vi "uv光源修改.vi"() -> ()   [LabVIEW 2018]
uses:
  <vilib>/Instr/_visa.llb/VISA Configure Serial Port (Instr).vi
panel:
  out "串口状态":bool
  out "错误输出":errorcluster
  in  "数值":u16
  in  "写入字符串":string="uvled"
  in  "光源强度":u16(ring) items=["5%", "10%", "15%", "20%", "25%", "30%", "40%", "45%", "50%", "55%", "60%", "65%", "70%", "75%", "80%", "85%", "90%", "95%", "100%", "开启光源", "关闭光源", "手动模式", "自动模式"]
  out "光源设置成功":bool
  in  "连接光源控制机":bool
  in  "发送":bool
  in  "停止":bool
  out "接收区":string
  out "连接成功":bool
  out "uv光源开启":bool
  out "uv光源关闭":bool
  in  "stop bits (10: 1 bit)":u16(ring)=10 caption="停止位（10: 1位）" items=["1.0"=10, "1.5"=15, "2.0"=20]
  in  "parity (0:none)":enum16{"None", "Odd", "Even", "Mark", "Space"}(ring) caption="奇偶（0:无）"
  in  "data bits (8)":u16=8 caption="数据比特(8)" min=5 max=8 step=1
  in  "baud rate (9600)":u32=9600 caption="波特率(9600)"
  in  "VISA resource name":refnum<visa-resource-name> caption="VISA资源名称"
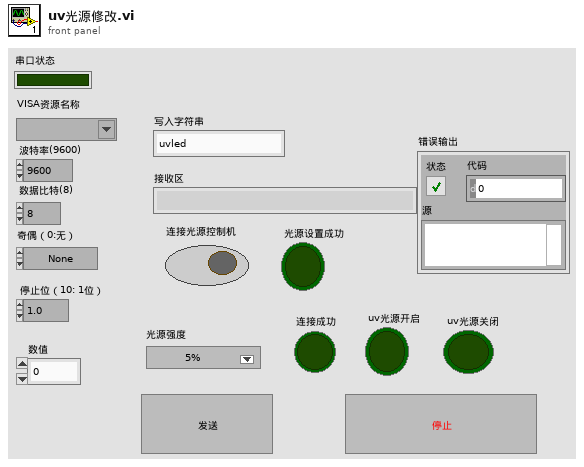
[diagram p1: front panel]
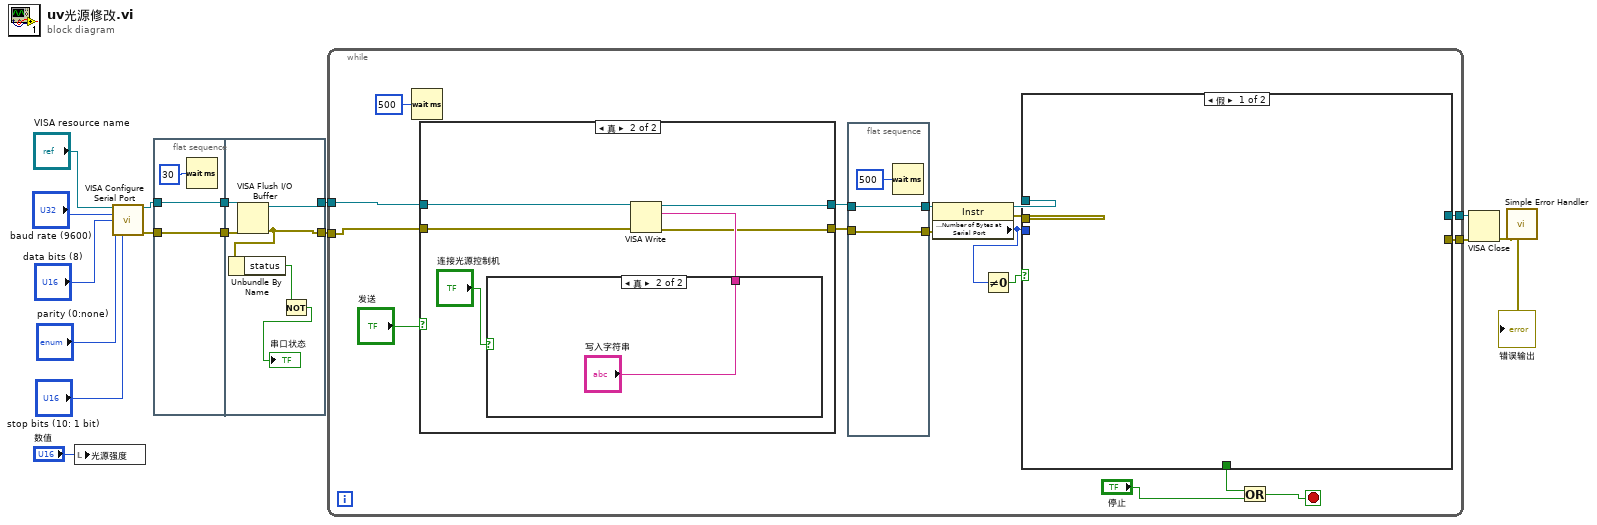
[diagram p0: block diagram]
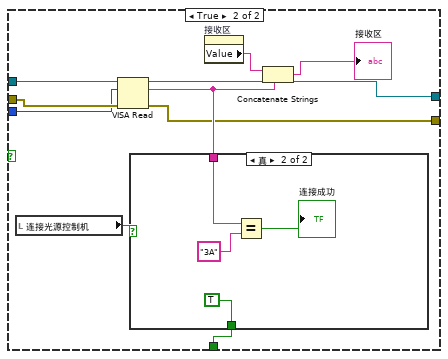
[diagram p2: hidden frame]
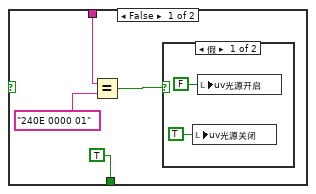
[diagram p3: hidden frame]
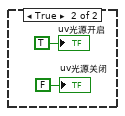
[diagram p4: hidden frame]
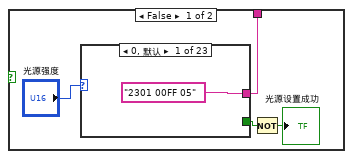
[diagram p6: hidden frame]
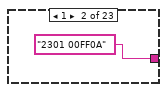
[diagram p7: hidden frame]
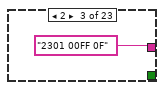
[diagram p8: hidden frame]
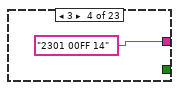
[diagram p9: hidden frame]
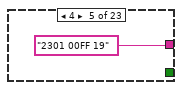
[diagram p10: hidden frame]
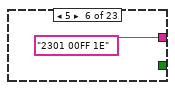
[diagram p11: hidden frame]
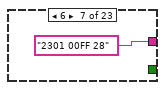
[diagram p12: hidden frame]
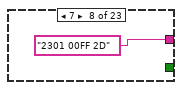
[diagram p13: hidden frame]
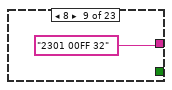
[diagram p14: hidden frame]
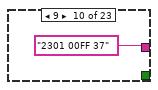
[diagram p15: hidden frame]
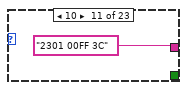
[diagram p16: hidden frame]
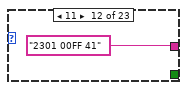
[diagram p17: hidden frame]
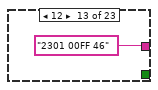
[diagram p18: hidden frame]
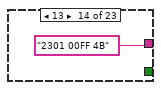
[diagram p19: hidden frame]
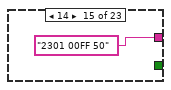
[diagram p20: hidden frame]
diagram:
  n1 = local write "光源强度"("数值") -> ()
  n2 = call-poly "VISA Configure Serial Port"("VISA resource name"="VISA resource name", "baud rate (9600)"="baud rate (9600)", "data bits (8)"="data bits (8)", "parity (0:none)"="parity (0:none)", "stop bits (10: 1 bit)"="stop bits (10: 1 bit)") -> ("VISA resource name out"=w4:refnum<visa-resource-name>, "error out"=w3:errorcluster)  [unwired: 9 in]
  n3 = flat-sequence {
    tunnel: w4 -> [w18]
    tunnel: w3 -> [w17]
    tunnel: [w18] -> w15
    tunnel: [w17] -> w14
    tunnel: [w21] -> w2
    tunnel: [w22] -> w1
    tunnel: w15 -> [w24]
    tunnel: w14 -> [w23]
    frame #0 {
      n4 = Wait (ms)(milliseconds to wait=u32 30 ("等待时间（毫秒）")) -> ()  [unwired: 1 out]
    }
    frame #1 {
      n5 = VISA Flush I/O Buffer(VISA resource name=w24, error in (no error)=w23) -> (VISA resource name out=w22:refnum<visa-resource-name>, error out=w21:errorcluster)  [unwired: 1 in]
      n6 = Unbundle By Name(w21) -> ("status"=w20:bool)
      n7 = Not(x=w20) -> (.not. x?=→"串口状态":bool)
    }
  }
  n8 = while {
    tunnel: w1 -> [w41]
    tunnel: [w29] -> w8
    tunnel: [w28] -> w6
    tunnel: w2 -> [w27]
    stop <- w32 stop-if-true
    n9 = Wait (ms)(milliseconds to wait=u32 500 ("等待时间（毫秒）")) -> ()  [unwired: 1 out]
    n10 = case shown="真" "发送" {
      tunnel: w41 -> [w67 w74]
      tunnel: w27 -> [w68 w73]
      tunnel: [w67 w71] -> w39
      tunnel: [w68 w70] -> w37
      frame False {
      }
      frame True {
        n11 = case shown="真" "连接光源控制机" {
          tunnel: [w78 "写入字符串"] -> w72
          frame False {
            n12 = case shown="0, 默认" "光源强度" {
              tunnel: ["2301 00FF 05" "2301 00FF0A" "2301 00FF 0F" "2301 00FF 14" "2301 00FF 19" "2301 00FF 1E" "2301 00FF 28" "2301 00FF 2D" "2301 00FF 32" "2301 00FF 37" "2301 00FF 3C" "2301 00FF 41" "2301 00FF 46" "2301 00FF 4B" "2301 00FF 50" "2301 00FF 55" "2301 00FF 5A" "2301 00FF 5F" "2301 00FF 64" "230E 0000 01" "230E 0000 00" "231E 00FF 03" "231E 00FF 01"] -> w78
              tunnel: [_ _ _ _ _ _ _ _ _ _ _ _ _ _ _ _ _ _ _ TRUE TRUE _ _] -> w76
              frame 0, Default {
              }
              frame 1 {
              }
              frame 2 {
              }
              frame 3 {
              }
              frame 4 {
              }
              frame 5 {
              }
              frame 6 {
              }
              frame 7 {
              }
              frame 8 {
              }
              frame 9 {
              }
              frame 10 {
              }
              frame 11 {
              }
              frame 12 {
              }
              frame 13 {
              }
              frame 14 {
              }
              frame 15 {
              }
              frame 16 {
              }
              frame 17 {
              }
              frame 18 {
              }
              frame 19 {
                # "开启光源"
              }
              frame 20 {
                # "关闭光源"
              }
              frame 21 {
                # "手动模式"
              }
              frame 22 {
                # "自动模式"
              }
            }
            n13 = Not(x=w76) -> (.not. x?=→"光源设置成功":bool)
          }
          frame True {
          }
        }
        n14 = VISA Write(VISA resource name=w74, write buffer=w72, error in (no error)=w73) -> (VISA resource name out=w71:refnum<visa-resource-name>, error out=w70:errorcluster)  [unwired: 1 out]
      }
    }
    n15 = flat-sequence {
      tunnel: w39 -> [w65]
      tunnel: [w65] -> w38
      tunnel: w37 -> [w64]
      tunnel: [w64] -> w36
      frame #0 {
        n16 = Wait (ms)(milliseconds to wait=u32 500 ("等待时间（毫秒）")) -> ()  [unwired: 1 out]
      }
    }
    n17 = property class="Instr"(reference=w38, error in=w36) -> (reference out=w34:refnum<visa-resource-name>, error out=w35:errorcluster, "Serial Settings:Number of Bytes at Serial Port"=w25:u32)
    n18 = Not Equal To 0?(x=w25) -> (x != 0?=w26:bool)
    n19 = case shown="假" w26 {
      tunnel: w35 -> [_ w51]
      tunnel: w34 -> [_ w50]
      tunnel: w25 -> [_ w49]
      tunnel: [_ w44] -> w31
      tunnel: [_ w43] -> w29
      tunnel: [_ w42] -> w28
      frame False {
      }
      frame True {
        n20 = local read "连接光源控制机"() -> (w46:bool)
        n21 = VISA Read(VISA resource name=w50, byte count=w49, error in (no error)=w51) -> (VISA resource name out=w42:refnum<visa-resource-name>, read buffer=w45:string, error out=w43:errorcluster)  [unwired: 1 out]
        n22 = case shown="真" w46 {
          tunnel: w45 -> [w55 w63]
          tunnel: [TRUE TRUE] -> w44
          frame False {
            n23 = Equal?(x=w55, y="240E 0000 01") -> (x = y?=w53:bool)
            n24 = case shown="假" w53 {
              frame False {
                n25 = local write "uv光源关闭"(TRUE ("uv光源关闭")) -> ()
                n26 = local write "uv光源开启"(FALSE ("uv光源开启")) -> ()
              }
              frame True {
                "uv光源开启" <- TRUE ("uv光源开启")
                "uv光源关闭" <- FALSE ("uv光源关闭")
              }
            }
          }
          frame True {
            n27 = Equal?(x=w63, y="3A") -> (x = y?=→"连接成功":bool)
          }
        }
        n28 = property on="接收区" class="Str"() -> ("Value"=w47:string)  [unwired: 2 in, 2 out]
        n29 = Concatenate Strings(w47, w45) -> (→"接收区":string)
      }
    }
    n30 = Or(x=w31, y="停止") -> (x .or. y?=w32:bool)
  }
  n31 = VISA Close(VISA resource name=w6, error in (no error)=w8) -> (error out=w7:errorcluster)
  "错误输出" <- w7
  n32 = call <vilib>:"Simple Error Handler.vi"("error in (no error)"=w7) -> ()  [unwired: 4 in, 5 out]
